vi "FB Global State.vi"(7 "operation":enum16{"read", "write"}(ring), 11 "State in":variant) -> (3 "State out":variant)   [LabVIEW 2020]
uses:
  <vilib>/functionblocks/FB Support/FB State.ctl
  <vilib>/BlockNodeSupport/BlockNodeState.ctl
  <vilib>/BlockNodeSupport/TerminalData.ctl
  <vilib>/picture/picture.llb/imagedata.ctl
  <vilib>/functionblocks/FB Support/FB User State.ctl
  <vilib>/functionblocks/FB Support/FB Polymorphic Data.ctl
  <vilib>/functionblocks/FB Support/FB Terminal Data.ctl
  <vilib>/functionblocks/FB Support/FB Terminal Source.ctl
  <vilib>/functionblocks/FB Support/FB Variable Data.ctl
  <vilib>/functionblocks/FB Support/FB Variable Access.ctl
  <vilib>/functionblocks/FB Support/FB Terminal Wired State.ctl
  <vilib>/functionblocks/FB Support/FB Flavor.ctl
  <vilib>/functionblocks/FB Support/FB Error Conditions.ctl
panel:
  in  "State":T1 {"BlockNodeState"."Draw Style" items=["FunctionBlock", "ExpressVI", "Variable", "Elemental I/O", "32x32 Icon", "FunctionBlockCompact"]; "BlockNodeState"."Terminal Data"."Terminal Flags" format="%.0b"}
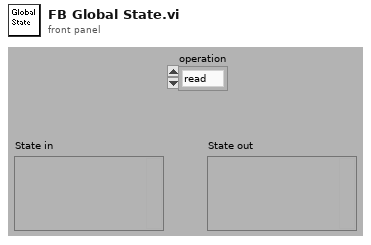
[diagram p1: front panel]
types:
  T1 = typedef "FB State.ctl" = cluster{"BlockNodeState":T2, "FB User State":T5}
  T2 = typedef "BlockNodeState.ctl" = cluster{"Terminal Data":T3[], "Instance Name":string, "Type Name":string, "Draw Style":i32, "Connector Pane Pattern":i32, "Flags":i32, "Grown Terminal List Order":i32[], "Image":T4}
  T3 = typedef "TerminalData.ctl" = cluster{"Terminal Name":string, "Terminal Display Name":string, "Terminal ID":string, "Terminal Flags":i32, "Terminal Type":variant, "Terminal Map ID":i32}
  T4 = typedef "imagedata.ctl" = cluster{"image type":i32, "image depth":i32, "image":u8[], "mask":u8[], "colors":u32[], "Rectangle":cluster{"left":i16, "top":i16, "right":i16, "bottom":i16}}
  T5 = typedef "FB User State.ctl" = cluster{"Poly VIs":T6[], "Folder Path":path, "Merge VI Path":path, "Poly VI Path":path, "Linker Source ID":string, "Poly Index":i32, "Modify Strings":string[], "Terminal Wired State":T11[], "Variant":variant, "Flavor":T12, "Error conditions":T13, "Bad Code?":bool}
  T6 = typedef "FB Polymorphic Data.ctl" = cluster{"Terminal Data":T7[], "VI Icon":T4, "Connector Pane Pattern":u32, "Source VI Path":path, "Variant":variant, "EN Terminal ID":string, "ENO Terminal ID":string, "Poly Instance VI Name":string}
  T7 = typedef "FB Terminal Data.ctl" = cluster{"Input Terminal?":bool, "Error Terminal?":bool, "Terminal Map ID":i32, "Terminal ID":string, "Terminal Configurable?":bool, "Long Display Name":string, "Short Display Name":string, "Terminal Default Value":variant, "Terminal Wire Rule":enum16{"Invalid Wire Rule", "Required", "Recommended", "Optional", "Dynamic Dispatch"}, "Data Source":T8, "Variable Data":T9, "Visible?":bool, "Typedef path":path}
  T8 = typedef "FB Terminal Source.ctl" = enum16{"Terminal", "Variable", "Default"}
  T9 = typedef "FB Variable Data.ctl" = cluster{"Variable name":string, "URL":string, "Variable scope":T10, "Variable data type":variant}
  T10 = typedef "FB Variable Access.ctl" = enum16{"Unsupported", "No Variable", "Single-process", "Network-published"}
  T11 = typedef "FB Terminal Wired State.ctl" = cluster{"Terminal ID":string, "Wired?":bool}
  T12 = typedef "FB Flavor.ctl" = enum16{"Function Block", "Function"}
  T13 = typedef "FB Error Conditions.ctl" = cluster{"No owning project":bool, "Permanently bad":bool}
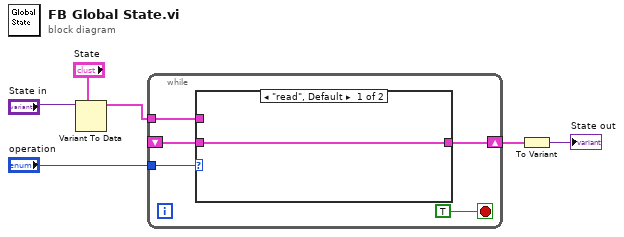
[diagram p0: block diagram]
diagram:
  n1 = Variant To Data(type="State", Variant="State in") -> (data=w3:T1)  [unwired: 1 in, 1 out]
  n2 = while {
    tunnel: w3 -> [w10]
    tunnel: "operation" -> [w9]
    shift-right: [w8] -> w2
    shift-left: _ -> [w7]
    stop <- TRUE stop-if-true
    n3 = case shown="\"read\", Default" w9 {
      tunnel: w10 -> [_ w13]
      tunnel: [w12 w13] -> w8
      tunnel: w7 -> [w12 _]
      frame "read", Default {
      }
      frame "write" {
      }
    }
  }
  n4 = To Variant(anything=w2) -> (Variant=→"State out":variant)
